vi "Main.vi"(11 "Module Admin":refnum<class "Delacor_lib_QMH_Module Admin.lvclass">) -> ()   [LabVIEW 2024, in "ControllerUI.lvlib"]
doc: "This template is based off of the Queued Message Handler design pattern and the Queued Message Handler project template that ships with LabVIEW.\n\nThe main difference is that the queue is private to this module and communication between modules is performed via Broadcast and Request events.\n\nRequest events are wrapped in public API methods and are handled in the Event Handling Loop (EHL) of this VI. Any module can register for Broadcast events sent by this module. The EHL generates messages based on user interface actions.\n\nThe Message Handling Loop (MHL) processes messages generated by the EHL, or by other messages. The messages are string values, so new messages can be added easily to the Message Cases case structure in the MHL. Each message cluster can also provide an optional value for Message Data, which is a variant that can be converted to whatever message-specific data is required.\n_____\nBased on DQMH Dev Tools: Project Template 7.1.0.1503."
uses:
  ControllerUI.lvlib
  <vilib>/Delacor/Delacor QMH/Libraries/Module Admin_class/Delacor_lib_QMH_Module Admin.lvclass
  Module Data--cluster.ctl
  <vilib>/Utility/miscctls.llb/LVFontTypeDef.ctl
  Stop Argument--cluster.ctl
  <vilib>/Delacor/Delacor QMH/Libraries/Message Queue_class/Delacor_lib_QMH_Message Queue.lvclass/Delacor_lib_QMH_Message Queue.ctl
  <vilib>/Delacor/Delacor QMH/Libraries/Module Admin_class/Delacor_lib_QMH_Module Admin.lvclass/Delacor_lib_QMH_Module Admin.ctl
  <vilib>/Delacor/Delacor QMH/Libraries/Message Queue_class/Delacor_lib_QMH_Enqueue Message (Single).vi
  <vilib>/Delacor/Delacor QMH/Libraries/Module Admin_class/Delacor_lib_QMH_Get External Launch.vi
  <vilib>/Delacor/Delacor QMH/Libraries/Message Queue_class/Delacor_lib_QMH_Message Queue.lvclass
  MoneyControl/MoneyControl.lvlib
  ProductControl/ProductControl.lvlib
  Mensajes/Mensajes.lvlib
panel:
  out "Status":string
  out "error out":errorcluster
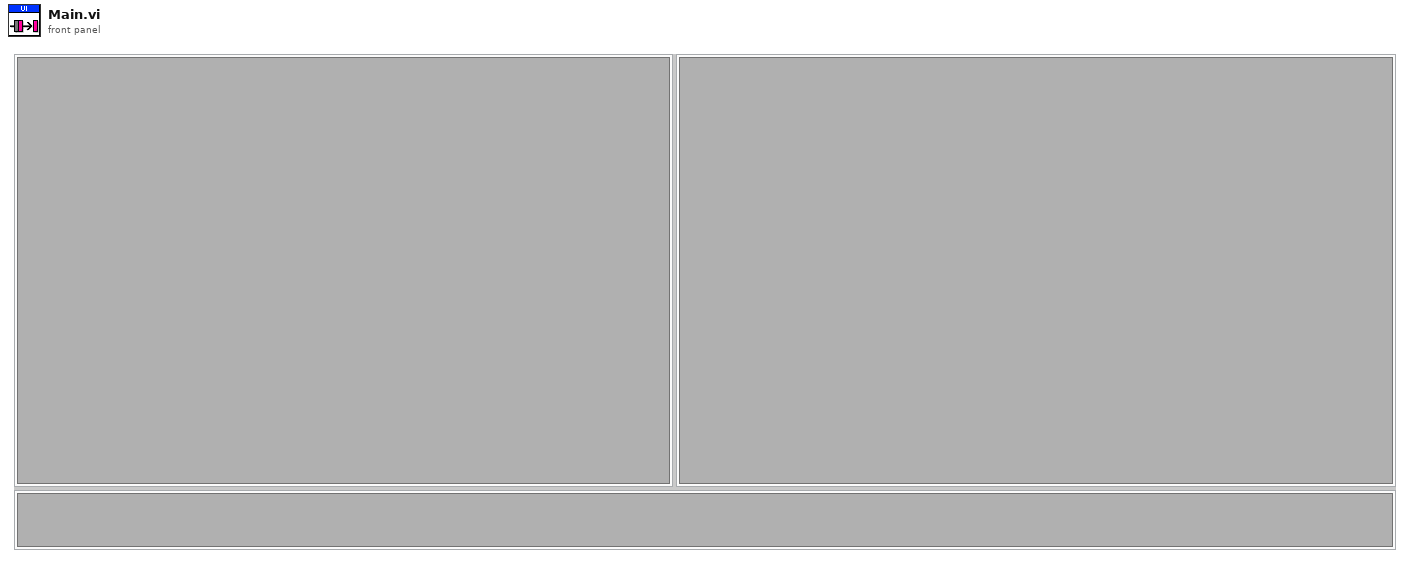
[diagram p1: front panel]
types:
  T1 = typedef "ControllerUI.lvlib/Request Events--cluster.ctl" = cluster{"Stop Module":refnum<user-event>, "Show Panel":refnum<user-event>, "Hide Panel":refnum<user-event>, "Get Module Execution Status":refnum<user-event>, "Show Diagram":refnum<user-event>}
  T2 = typedef "MoneyControl.lvlib/Broadcast Events--cluster.ctl" = cluster{"Module Did Init":refnum<user-event>, "Status Updated":refnum<user-event>, "Error Reported":refnum<user-event>, "Module Did Stop":refnum<user-event>, "Update Module Execution Status":refnum<user-event>}
  T3 = typedef "ProductControl.lvlib/Broadcast Events--cluster.ctl" = cluster{"Module Did Init":refnum<user-event>, "Status Updated":refnum<user-event>, "Error Reported":refnum<user-event>, "Module Did Stop":refnum<user-event>, "Update Module Execution Status":refnum<user-event>}
  T4 = typedef "Mensajes.lvlib/Broadcast Events--cluster.ctl" = cluster{"Module Did Init":refnum<user-event>, "Status Updated":refnum<user-event>, "Error Reported":refnum<user-event>, "Module Did Stop":refnum<user-event>, "Update Module Execution Status":refnum<user-event>}
  T5 = typedef "ControllerUI.lvlib/Module Data--cluster.ctl" = cluster{"Status":string}
  T6 = typedef "LVFontTypeDef.ctl" = cluster{"Font Name":string, "Size":u16, "Bold":bool, "Italic":bool, "Underline":bool, "Strikeout":bool, "Color":u32}
  T7 = enum32{"invalid lock state", "Not Locked", "Locked (No Password)", "Password-protected"}
  T8 = typedef "ControllerUI.lvlib/Stop Argument--cluster.ctl" = cluster{"Origin":string, "Exit via Stop Module Req?":bool, "Wait for Module to stop?":bool}
  T9 = enum32{"Invalid", "Standard", "Closed", "Hidden", "Minimized", "Maximized"}
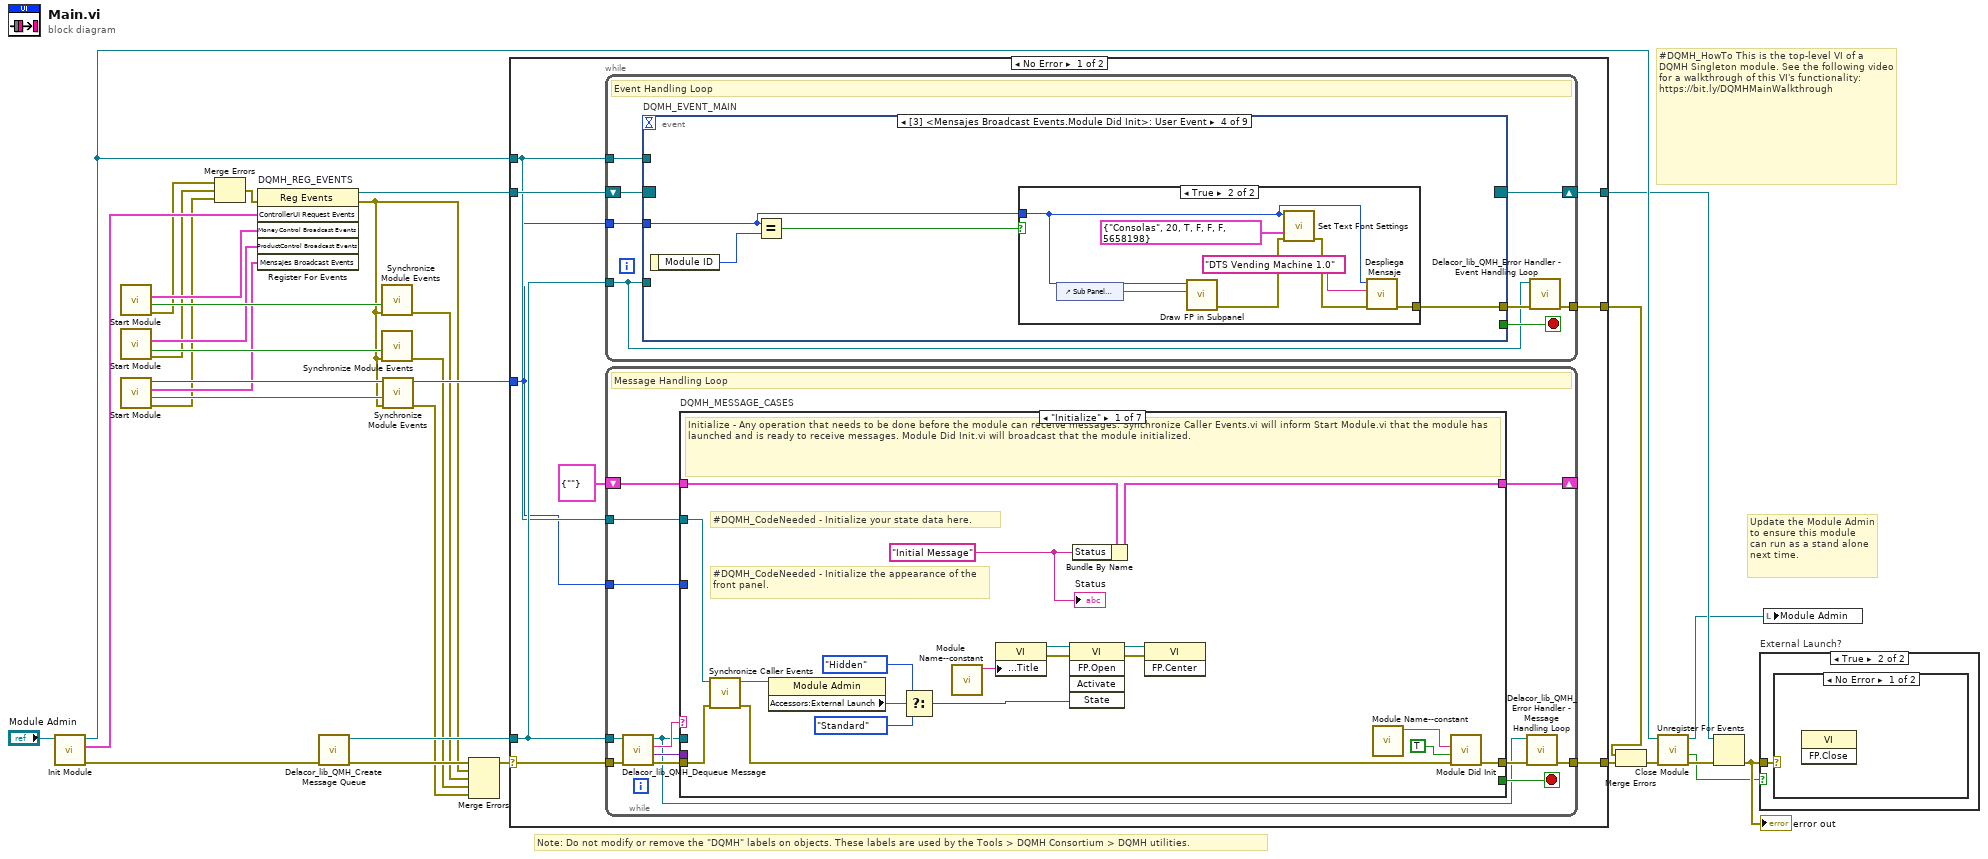
[diagram p0: block diagram]
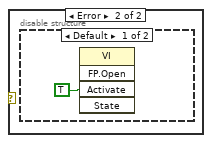
[diagram p3: hidden frame]
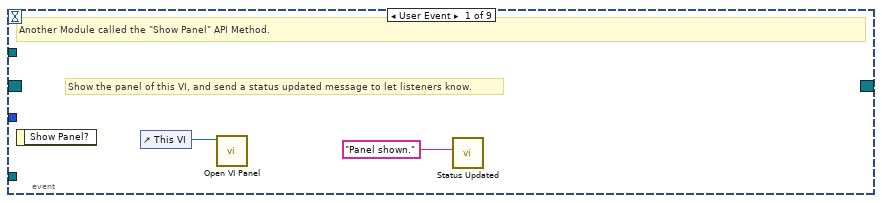
[diagram p5: hidden frame]
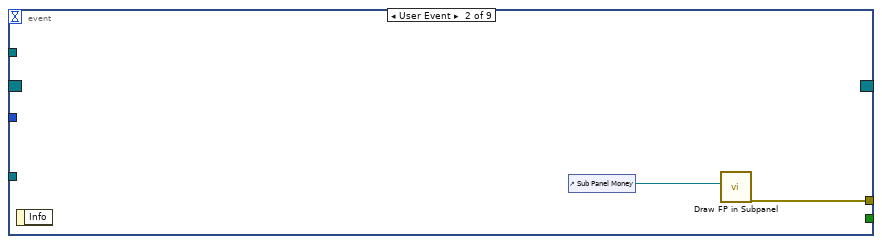
[diagram p6: hidden frame]
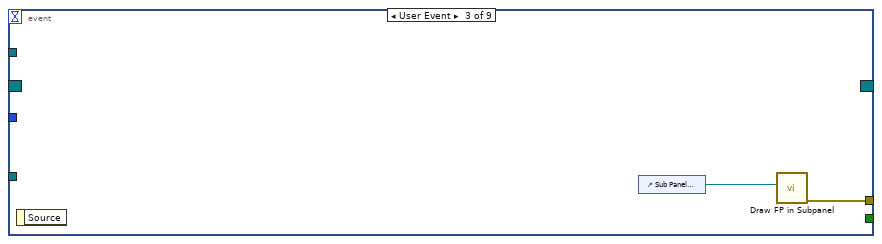
[diagram p7: hidden frame]
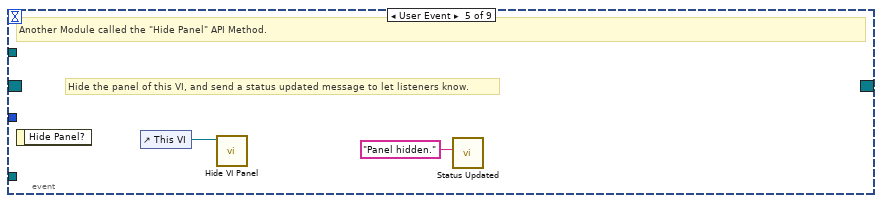
[diagram p9: hidden frame]
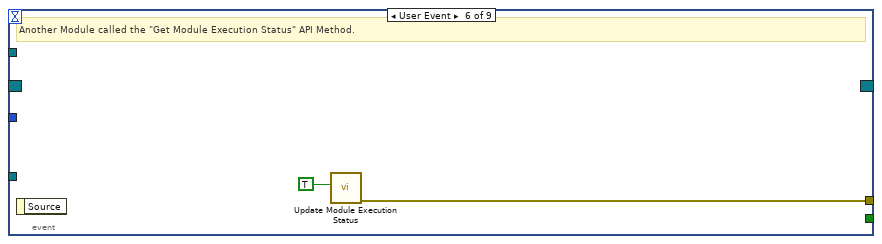
[diagram p10: hidden frame]
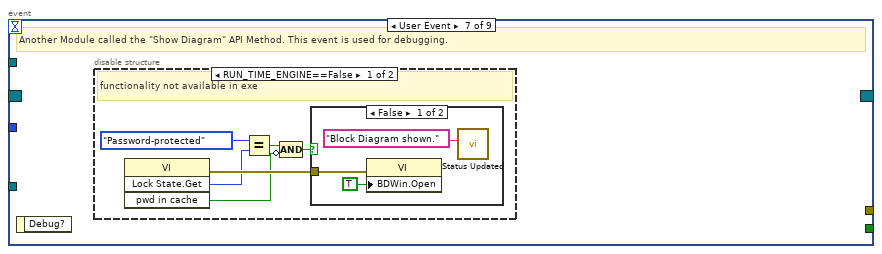
[diagram p11: hidden frame]
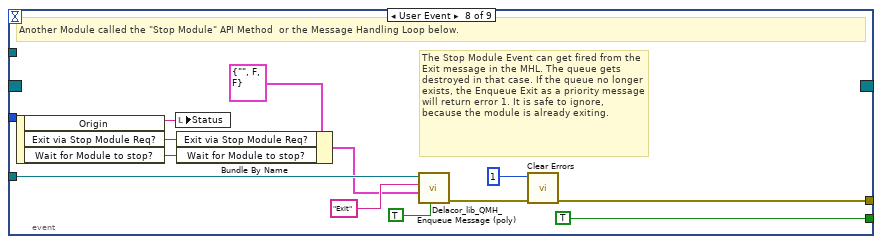
[diagram p14: hidden frame]
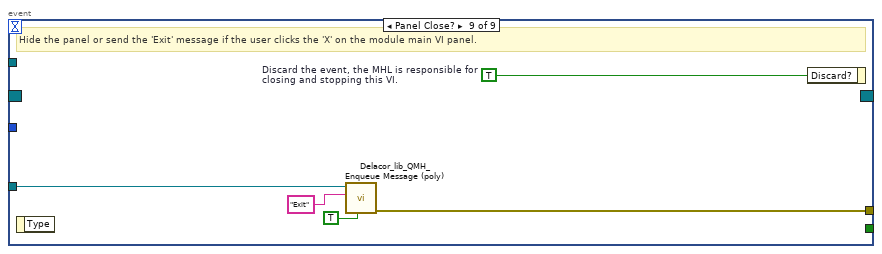
[diagram p15: hidden frame]
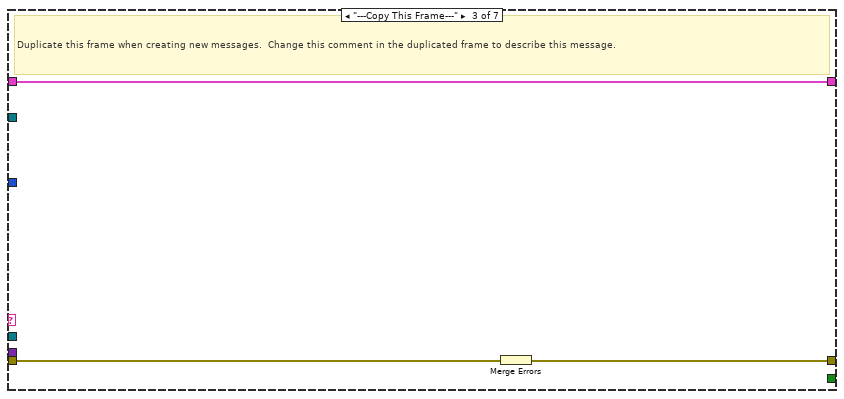
[diagram p17: hidden frame]
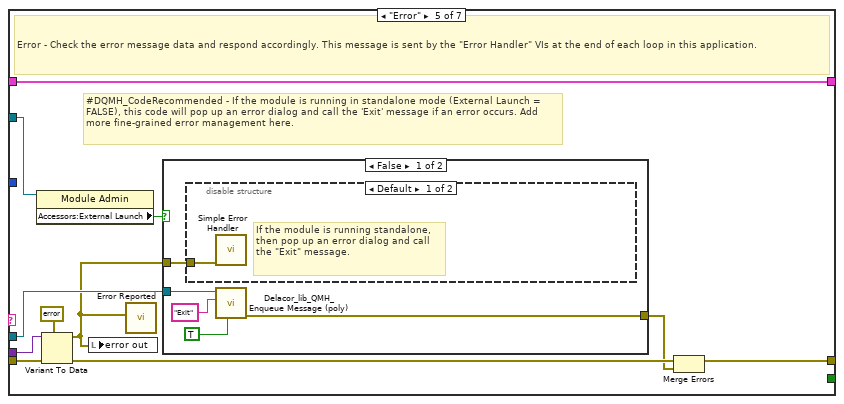
[diagram p19: hidden frame]
diagram:
  # "#DQMH_HowTo This is the top-level VI of a DQMH Singleton module. See the following video for a walkthrough of this VI's functionality: https://bit.ly/DQMHMainWalkthrough"
  # "Note: Do not modify or remove the \"DQMH\" labels on objects. These labels are used by the Tools > DQMH Consortium > DQMH utilities."
  # "Update the Module Admin to ensure this module can run as a stand alone next time."
  n1 = call "Init Module.vi"("Singleton Module Admin in"="Module Admin") -> ("error out"=w31:errorcluster, "ControllerUI Request Events"=w21:T1, "Singleton Module Admin out"=w24:refnum<class "Delacor_lib_QMH_Module Admin.lvclass">)  [unwired: 8 in]
  n2 = call "Start Module.vi"() -> ("error out"=w6:errorcluster, "Wait for Event Sync?"=w15:bool, "MoneyControl Broadcast Events"=w16:T2)  [unwired: 7 in, 2 out]
  n3 = call "Start Module.vi"() -> ("error out"=w5:errorcluster, "Wait for Event Sync?"=w14:bool, "ProductControl Broadcast Events"=w13:T3)  [unwired: 7 in, 2 out]
  n4 = call "Start Module.vi"() -> ("error out"=w4:errorcluster, "Wait for Event Sync?"=w11:bool, "Mensajes Broadcast Events"=w10:T4, "Module ID"=w12:i32)  [unwired: 7 in, 1 out]
  n5 = Merge Errors(w6, w5, w4) -> (w7:errorcluster)
  n6 = register-events "DQMH_REG_EVENTS"(error in=w7, w21, w16, w13, w10) -> (reference out=w22:refnum<event-registration>, error out=w8:errorcluster)  [unwired: 1 in]
  n7 = call <vilib>:"Delacor_lib_QMH_Create Message Queue.vi"("error in"=w31) -> ("error out"=w26:errorcluster, "Message Queue"=w20:refnum<class "Delacor_lib_QMH_Message Queue.lvclass">)  [unwired: 9 in]
  n8 = call "Synchronize Module Events.vi"("error in"=w8, "Wait for Event Sync?"=w15) -> ("error out"=w3:errorcluster)  [unwired: 9 in]
  n9 = call "Synchronize Module Events.vi"("error in"=w8, "Wait for Event Sync?"=w14) -> ("error out"=w2:errorcluster)  [unwired: 9 in]
  n10 = call "Synchronize Module Events.vi"("error in"=w8, "Wait for Event Sync?"=w11, "Module ID in"=w12) -> ("error out"=w1:errorcluster, "Module ID out"=w9:i32)  [unwired: 7 in]
  n11 = Merge Errors(w26, w8, w3, w2, w1) -> (w25:errorcluster)
  n12 = case shown="No Error" w25 {
    selector: w25 -> [w39 w187]
    tunnel: [w41 w186] -> w32
    tunnel: [w38 w185] -> w23
    tunnel: w22 -> [w36 w185]
    tunnel: w20 -> [w35 w181]
    tunnel: [w40 _] -> w29
    tunnel: w24 -> [w34 w182]
    tunnel: w9 -> [w33 w180]
    frame No Error {
      n13 = while {
        tunnel: w35 -> [w43]
        shift-right: [w46] -> w38
        shift-left: w36 -> [w47]
        tunnel: [w48] -> w40
        tunnel: w34 -> [w44]
        tunnel: w33 -> [w42]
        stop <- w45 stop-if-true
        # "Event Handling Loop"
        n14 = event "DQMH_EVENT_MAIN" shown="[3] <Mensajes Broadcast Events.Module Did Init>: User Event" {
          selector: w47 -> [_ _ _ _ _ _ _ _ _]
          dyn-events: [_ _ _ _ _ _ _ _ _] -> w46
          timeout: _ -> [_ _ _ _ _ _ _ _ _]
          tunnel: [_ _ _ _ _ _ _ TRUE ("Discard?") _] -> w45
          tunnel: w43 -> [_ _ _ _ _ _ _ w87 w94]
          tunnel: [_ w52 w55 w59 _ w70 _ w90 w96] -> w49
          tunnel: w44 -> [_ _ _ _ _ _ _ _ _]
          tunnel: w42 -> [_ _ _ w56 _ _ _ _ _]
          event User Event {
            # "Show the panel of this VI, and send a status updated message to let listeners know."
            # "Another Module called the \"Show Panel\" API Method."
            n15 = event-data() -> ()  [unwired: 1 in, 1 out]
            n16 = control-ref of="This VI"() -> (w51:refnum<vi>)
            n17 = call "Open VI Panel.vi"("VI"=w51) -> ()  [unwired: 10 in, 1 out]
            n18 = call "Status Updated.vi"("Status"="Panel shown." ("format string")) -> ()  [unwired: 10 in, 1 out]
          }
          event User Event {
            n19 = event-data() -> ()  [unwired: 1 in, 1 out]
            n20 = control-ref of="Sub Panel Money"() -> (w53:refnum<vi>)
            n21 = call "Draw FP in Subpanel.vi"("Sub Panel"=w53) -> ("error out"=w52:errorcluster)  [unwired: 10 in]
          }
          event User Event {
            n22 = event-data() -> ()  [unwired: 1 in, 1 out]
            n23 = control-ref of="Sub Panel Products"() -> (w54:refnum<vi>)
            n24 = call "Draw FP in Subpanel.vi"("Sub Panel"=w54) -> ("error out"=w55:errorcluster)  [unwired: 10 in]
          }
          event User Event {
            n25 = event-data() -> ("Module ID"=w58:i32)  [unwired: 1 in]
            n26 = Equal?(x=w56, y=w58) -> (x = y?=w57:bool)
            n27 = case shown="True" w57 {
              tunnel: [_ w62] -> w59
              tunnel: w56 -> [_ w61]
              frame False {
              }
              frame True {
                n28 = control-ref of="Sub Panel Mensajes"() -> (w66:refnum<vi>)
                n29 = call "Draw FP in Subpanel.vi"("Sub Panel"=w66, "Module ID"=w61) -> ("error out"=w65:errorcluster)  [unwired: 9 in]
                n30 = call "Set Text Font Settings.vi"("error in"=w65, "Text.Font"=T6 {"Font Name"="Consolas", "Size"=20, "Bold"=TRUE, "Italic"=FALSE, "Underline"=FALSE, "Strikeout"=FALSE, "Color"=5658198}, "Module ID"=w61) -> ("error out"=w63:errorcluster)  [unwired: 8 in]
                n31 = call "Despliega Mensaje.vi"("error in"=w63, "Mensaje"="DTS Vending Machine 1.0", "Module ID"=w61) -> ("error out"=w62:errorcluster)  [unwired: 8 in]
              }
            }
          }
          event User Event {
            # "Hide the panel of this VI, and send a status updated message to let listeners know."
            # "Another Module called the \"Hide Panel\" API Method."
            n32 = event-data() -> ()  [unwired: 1 in, 1 out]
            n33 = control-ref of="This VI"() -> (w68:refnum<vi>)
            n34 = call "Hide VI Panel.vi"("VI"=w68) -> ()  [unwired: 10 in, 1 out]
            n35 = call "Status Updated.vi"("Status"="Panel hidden." ("format string")) -> ()  [unwired: 10 in, 1 out]
          }
          event User Event {
            # "Another Module called the \"Get Module Execution Status\" API Method."
            n36 = event-data() -> ()  [unwired: 1 in, 1 out]
            n37 = call "Update Module Execution Status.vi"("Running?"=TRUE) -> ("error out"=w70:errorcluster)  [unwired: 10 in]
          }
          event User Event {
            # "Another Module called the \"Show Diagram\" API Method. This event is used for debugging."
            n38 = event-data() -> ()  [unwired: 1 in, 1 out]
            n39 = disable-structure shown="RUN_TIME_ENGINE==False" {
              frame condition #0 (active) {
                # "functionality not available in exe"
                n40 = invoke on="Invoke Node" class="VI" method="Lock State.Get"() -> (error out=w76:errorcluster, "Get Lock State"=w75:T7, "pwd in cache"=w72:bool)  [unwired: 4 in, 1 out]
                n41 = Equal?(x=T7."Password-protected", y=w75) -> (x = y?=w73:bool)
                n42 = Compound Arithmetic op=AND(w73, invert w72) -> (w71:bool)
                n43 = case shown="False" w71 {
                  tunnel: w76 -> [w79 _]
                  frame False {
                    n44 = property on="Property Node" class="VI"(error in=w79, "BDWin.Open"=TRUE ("Block Diagram Window:Open")) -> ()  [unwired: 1 in, 2 out]
                    n45 = call "Status Updated.vi"("Status"="Block Diagram shown." ("format string")) -> ()  [unwired: 10 in, 1 out]
                  }
                  frame True {
                    # "Password-protected VI, and the password is not in the cache. Do not show the diagram."
                  }
                }
              }
              frame condition #1 {
              }
            }
          }
          event User Event {
            # "The Stop Module Event can get fired from the Exit message in the MHL. The queue gets destroyed in that case. If the queue no longer exists, the Enqueue Exit as a priority message will return error 1. It is safe to ignore, because the module is already exiting."
            # "Another Module called the \"Stop Module\" API Method  or the Message Handling Loop below."
            n46 = event-data() -> ("Origin"=w86:string, "Exit via Stop Module Req?"=w82:bool, "Wait for Module to stop?"=w81:bool)  [unwired: 1 in]
            n47 = local write "Status"(w86) -> ()
            n48 = Bundle By Name(cluster=T8 {"Origin"="", "Exit via Stop Module Req?"=FALSE, "Wait for Module to stop?"=FALSE} ("Stop Argument"), "Exit via Stop Module Req?"=w82, "Wait for Module to stop?"=w81) -> (w80:T8)
            n49 = call-poly <vilib>:"Delacor_lib_QMH_Enqueue Message (poly).vi"("Priority Message? (F)"=TRUE, "Message Data"=w80, "Message"="Exit", "Message Queue in"=w87) -> ("error out"=w91:errorcluster)  [unwired: 6 in, 1 out]
            n50 = call <vilib>:"Clear Errors.vi"("error in (no error)"=w91, "specific error code to clear (0: all)"=1) -> ("error out"=w90:errorcluster)  [unwired: 4 in, 1 out]
          }
          event Panel Close? {
            w95 = TRUE  # Discard the event, the MHL is responsible for closing and stopping this VI.
            # "Hide the panel or send the 'Exit' message if the user clicks the 'X' on the module main VI panel."
            n51 = event-data() -> ()  [unwired: 1 in, 1 out]
            n52 = call-poly <vilib>:"Delacor_lib_QMH_Enqueue Message (poly).vi"("Priority Message? (F)"=TRUE, "Message"="Exit", "Message Queue in"=w94) -> ("error out"=w96:errorcluster)  [unwired: 7 in, 1 out]
            n53 = event-data ("Event Filter Node")("Discard?"=w95) -> ()  [unwired: 1 in, 1 out]
          }
        }
        n54 = call-dynamic "Delacor_lib_QMH_Error Handler - Event Handling Loop.vi"("error in"=w49, "Message Queue in"=w43) -> ("dup error in"=w48:errorcluster)  [unwired: 8 in, 1 out]
      }
      n55 = while {
        tunnel: w35 -> [w98]
        shift-right: [w106] -> _
        shift-left: T5 {"Status"=""} ("Data Cluster") -> [w107]
        tunnel: w39 -> [w109]
        tunnel: [w101] -> w41
        tunnel: w34 -> [w102]
        tunnel: w33 -> [w97]
        stop <- w105 stop-if-true
        # "Message Handling Loop"
        n56 = call-dynamic "Delacor_lib_QMH_Dequeue Message.vi"("error in"=w109, "Message Queue in"=w98) -> ("error out"=w108:errorcluster, "Message Data"=w103:variant, "Message"=w104:string, "Message Queue out"=w99:refnum<class "Delacor_lib_QMH_Message Queue.lvclass">)  [unwired: 6 in]
        n57 = case "DQMH_MESSAGE_CASES" shown="\"Initialize\"" w104 {
          selector: w104 -> [_ _ _ _ _ _ w174]
          tunnel: w99 -> [_ _ _ _ w139 w162 _]
          tunnel: w108 -> [w126 w130 w133 w135 w146 w168 w177]
          tunnel: [w124 w130 w132 w135 w142 w163 w178] -> w100
          tunnel: w107 -> [w115 w129 w131 w134 w141 w161 w175]
          tunnel: [w114 w129 w131 w134 w141 w161 w175] -> w106
          tunnel: [_ _ _ _ _ w160 _] -> w105
          tunnel: w103 -> [_ _ _ _ w140 w159 _]
          tunnel: w102 -> [w116 _ _ _ w138 w154 _]
          tunnel: w97 -> [_ _ _ _ _ w153 _]
          frame "Initialize" {
            w110 = "Initial Message" ("Initial Message")
            # "#DQMH_CodeNeeded - Initialize the appearance of the front panel."
            # "#DQMH_CodeNeeded - Initialize your state data here."
            # "Initialize - Any operation that needs to be done before the module can receive messages. Synchronize Caller Events.vi will inform Start Module.vi that the module has launched and is ready to receive messages. Module Did Init.vi will broadcast that the module initialized."
            n58 = call "Synchronize Caller Events.vi"("error in"=w126, "Singleton Module Admin in"=w116) -> ("error out"=w125:errorcluster, "Singleton Module Admin out"=w111:refnum<class "Delacor_lib_QMH_Module Admin.lvclass">)  [unwired: 8 in]
            n59 = property on="Property Node" class="Module Admin"(reference=w111) -> ("Accessors:External Launch"=w120:bool)  [unwired: 1 in, 2 out]
            n60 = Select(t=T9."Hidden" ("State"), s=w120, f=T9."Standard" ("State")) -> (s? t:f=w117:T9)
            n61 = call "Module Name--constant.vi"() -> ("Module Name"=w123:string)  [unwired: 11 in]
            n62 = property on="Property Node" class="VI"("Front Panel.Title"=w123) -> (reference out=w122:refnum<vi>, error out=w128:errorcluster)  [unwired: 2 in]
            n63 = invoke on="Invoke Node" class="VI" method="FP.Open"(reference=w122, error in=w128, "State"=w117) -> (reference out=w121:refnum<vi>, error out=w127:errorcluster)  [unwired: 2 in, 3 out]
            n64 = Bundle By Name(cluster=w115, "Status"=w110) -> (w114:T5)
            n65 = invoke on="Invoke Node" class="VI" method="FP.Center"(reference=w121, error in=w127) -> ()  [unwired: 1 in, 3 out]
            n66 = call "Module Name--constant.vi"() -> ("Module Name"=w112:string)  [unwired: 11 in]
            n67 = call "Module Did Init.vi"("error in"=w125, "Initialized?"=TRUE, "Origin"=w112) -> ("error out"=w124:errorcluster)  [unwired: 8 in]
            "Status" <- w110
          }
          frame "---Module Specific---" {
            # "Separator -- The following cases handle messages specific to this Module."
          }
          frame "---Copy This Frame---" {
            # "Duplicate this frame when creating new messages.  Change this comment in the duplicated frame to describe this message."
            n68 = Merge Errors(w133) -> (w132:errorcluster)
          }
          frame "---Exit and Error Handling---" {
            # "Separator - The following cases handle errors and exit messages."
          }
          frame "Error" {
            # "#DQMH_CodeRecommended - If the module is running in standalone mode (External Launch = FALSE), this code will pop up an error dialog and call the 'Exit' message if an error occurs. Add more fine-grained error management here."
            # "Error - Check the error message data and respond accordingly. This message is sent by the \"Error Handler\" VIs at the end of each loop in this application."
            n69 = property on="Property Node" class="Module Admin"(reference=w138) -> ("Accessors:External Launch"=w137:bool)  [unwired: 1 in, 2 out]
            n70 = Variant To Data(error in=w146, type=errorcluster {"status"=FALSE, "code"=0, "source"=""} ("error constant"), Variant=w140) -> (data=w136:errorcluster, error out=w144:errorcluster)
            n71 = local write "error out"(w136) -> ()
            n72 = call "Error Reported.vi"("Error"=w136) -> ()  [unwired: 10 in, 1 out]
            n73 = case shown="False" w137 {
              tunnel: [w151 _] -> w143
              tunnel: w139 -> [w149 _]
              tunnel: w136 -> [w150 _]
              frame False {
                n74 = disable-structure shown="Default" {
                  disable-tunnel: w150 -> [w152 _]
                  frame condition #0 (active) {
                    # "If the module is running standalone, then pop up an error dialog and call the \"Exit\" message."
                    n75 = call <vilib>:"Simple Error Handler.vi"("error in (no error)"=w152) -> ()  [unwired: 4 in, 5 out]
                  }
                  frame condition #1 {
                    # "To prevent the Simple Error Handler VI from being loaded (e.g. when deploying to a Real-Time target), add the Conditional Disable Symbol \"DQMH_Disable_SEH\" to your project and set it to TRUE."
                  }
                }
                n76 = call-poly <vilib>:"Delacor_lib_QMH_Enqueue Message (poly).vi"("Priority Message? (F)"=TRUE, "Message"="Exit", "Message Queue in"=w149) -> ("error out"=w151:errorcluster)  [unwired: 7 in, 1 out]
              }
              frame True {
                # "If the module was launched externally, calling the Error Reported broadcast VI is the only action performed by the \"Error\" message. The module's caller can then process the error appropriately."
              }
            }
            n77 = Merge Errors(w144, w143) -> (w142:errorcluster)
          }
          frame "Exit" {
            w158 = 91  # 91: not all Exit messages will have an argument
            w160 = TRUE  # Stop the VI
            # "Release the message queue reference"
            # "Exit - Exit the application."
            n78 = Variant To Data(error in=w168, type=T8 {"Origin"="", "Exit via Stop Module Req?"=FALSE, "Wait for Module to stop?"=FALSE} ("Stop Argument"), Variant=w159) -> (data=w156:T8, error out=w165:errorcluster)
            n79 = call <vilib>:"Clear Errors.vi"("error in (no error)"=w165, "specific error code to clear (0: all)"=w158) -> ("error out"=w167:errorcluster)  [unwired: 4 in, 1 out]
            n80 = control-ref of="This VI"() -> (w155:refnum<vi>)
            n81 = call-dynamic "Delacor_lib_QMH_Release Message Queue.vi"("error in"=w167, "Message Queue"=w162) -> ("error out"=w166:errorcluster)  [unwired: 9 in]
            n82 = call "Handle Exit.vi"("Stop Argument"=w156, "Admin in"=w154, "VI reference"=w155) -> ("error out"=w164:errorcluster)  [unwired: 7 in, 1 out]
            n83 = Merge Errors(w166, w164) -> (w163:errorcluster)
            n84 = call "Error Reported.vi"("Error"=w163) -> ()  [unwired: 10 in, 1 out]
            n85 = call "Stop Module.vi"() -> ()  [unwired: 11 in, 1 out]
            n86 = call "Stop Module.vi"() -> ()  [unwired: 11 in, 1 out]
            n87 = call "Stop Module.vi"("Module ID"=w153) -> ()  [unwired: 10 in, 1 out]
          }
          frame Default {
            # "'Default' case only runs if there is a message that isn't defined in any of the other cases.  Output a programming error."
            n88 = call "Module Name--constant.vi"() -> ("Module Name"=w173:string)  [unwired: 11 in]
            n89 = Format Into String(format string="The invalid message string \"%s\" was received in the Message Handling Loop for module \"%s\".", w174, w173) -> (resulting string=w169:string)  [unwired: 2 in, 1 out]
            n90 = call <vilib>:"Error Cluster From Error Code.vi"("show call chain? (False)"=TRUE, "error message (\"\")"=w169, "error code (0)"=1) -> ("error out"=w176:errorcluster)  [unwired: 6 in]
            n91 = Merge Errors(w177, w176) -> (w178:errorcluster)
          }
        }
        n92 = call-dynamic "Delacor_lib_QMH_Error Handler - Message Handling Loop.vi"("error in"=w100, "Message Queue in"=w99) -> ("dup error in"=w101:errorcluster)  [unwired: 8 in, 1 out]
      }
    }
    frame Error {
      # "Synchronize Caller Events.vi will inform Start Module.vi that the module has launched and will let the code calling Start Module.vi register for broadcasts and would permit the caller receive the broadcast that an error occurred at launch time."
      n93 = call-dynamic "Delacor_lib_QMH_Release Message Queue.vi"("error in"=w187, "Message Queue"=w181) -> ("error out"=w186:errorcluster)  [unwired: 9 in]
      n94 = call "Synchronize Caller Events.vi"("Singleton Module Admin in"=w182) -> ("error out"=w188:errorcluster)  [unwired: 9 in, 1 out]
      n95 = call "Module Name--constant.vi"() -> ("Module Name"=w184:string)  [unwired: 11 in]
      n96 = Format Into String(format string="An error occurred during initialization. %s is no longer running.", w184) -> (resulting string=w179:string)  [unwired: 2 in, 1 out]
      n97 = Merge Errors(w186, w188) -> (w189:errorcluster)
      n98 = call "Error Reported.vi"("Additional Information"=w179, "Error"=w189) -> ()  [unwired: 9 in, 1 out]
      n99 = call "Stop Module.vi"("Origin"=w179) -> ()  [unwired: 10 in, 1 out]
      n100 = call "Stop Module.vi"("Origin"=w179, "Module ID"=w180) -> ()  [unwired: 9 in, 1 out]
      n101 = call "Stop Module.vi"("Origin"=w179) -> ()  [unwired: 10 in, 1 out]
    }
  }
  n102 = Merge Errors(w29, w32) -> (w28:errorcluster)
  n103 = call "Close Module.vi"("error in"=w28, "Module Admin in"=w24) -> ("error out"=w30:errorcluster, "External Launch"=w17:bool, "Module Admin out"=w18:refnum<class "Delacor_lib_QMH_Module Admin.lvclass">)  [unwired: 7 in]
  n104 = Unregister For Events(event registration refnum=w23, error in=w30) -> (error out=w27:errorcluster)
  "error out" <- w27
  n105 = case "External Launch?" shown="True" w17 {
    tunnel: w27 -> [_ w190]
    frame False {
    }
    frame True {
      n106 = case shown="No Error" w190 {
        frame No Error {
          n107 = invoke on="Invoke Node" class="VI" method="FP.Close"() -> ()  [unwired: 3 in, 3 out]
        }
        frame Error {
          n108 = disable-structure shown="Default" {
            frame condition #0 (active) {
              n109 = invoke class="VI" method="FP.Open"("Activate"=TRUE ("Activate?")) -> ()  [unwired: 4 in, 5 out]
            }
            frame condition #1 {
              # "Don't show panel on error if running inside a built EXE."
            }
          }
        }
      }
    }
  }
  n110 = local write "Module Admin"(w18) -> ()
